vi "Align with Gear Peg.vi"(0 "Targets Message":T5={"type"="", "message"={"capturedAgoMs"=0, "targets"=[{"x"=0.0, "y"=0.0, "z"=0.0, "theta"=0.0}]}}, 1 "Swerve DevRef":T1[](array[typedef]), 2 "Wheel DevRef":T1[](array[typedef]), 3 "error in":errorcluster) -> (4 "Wheel Speed":dbl[](array[numeric]), 5 "Reverse?":bool[](array[boolean]), 6 "Swerve Speed":dbl[](array[numeric]), 7 "Setpoint":dbl[](array[numeric]), 8 "error out":errorcluster)   [LabVIEW 2016]
uses:
  Vision/Messages/Targets/Targets Message.ctl
  Vision/Messages/Targets/Targets Info.ctl
  <vilib>/Rock Robotics/WPI/MotorControl/WPI_MotorControlDeviceRef.ctl
  <vilib>/Rock Robotics/WPI/MotorControl/WPI_MotorControlType.ctl
  <vilib>/Rock Robotics/SystemInterfaces/DIO/FPGA_DIOPWMChannel.ctl
  <vilib>/Rock Robotics/WPI/PWM/WPI_PWMDeadband.ctl
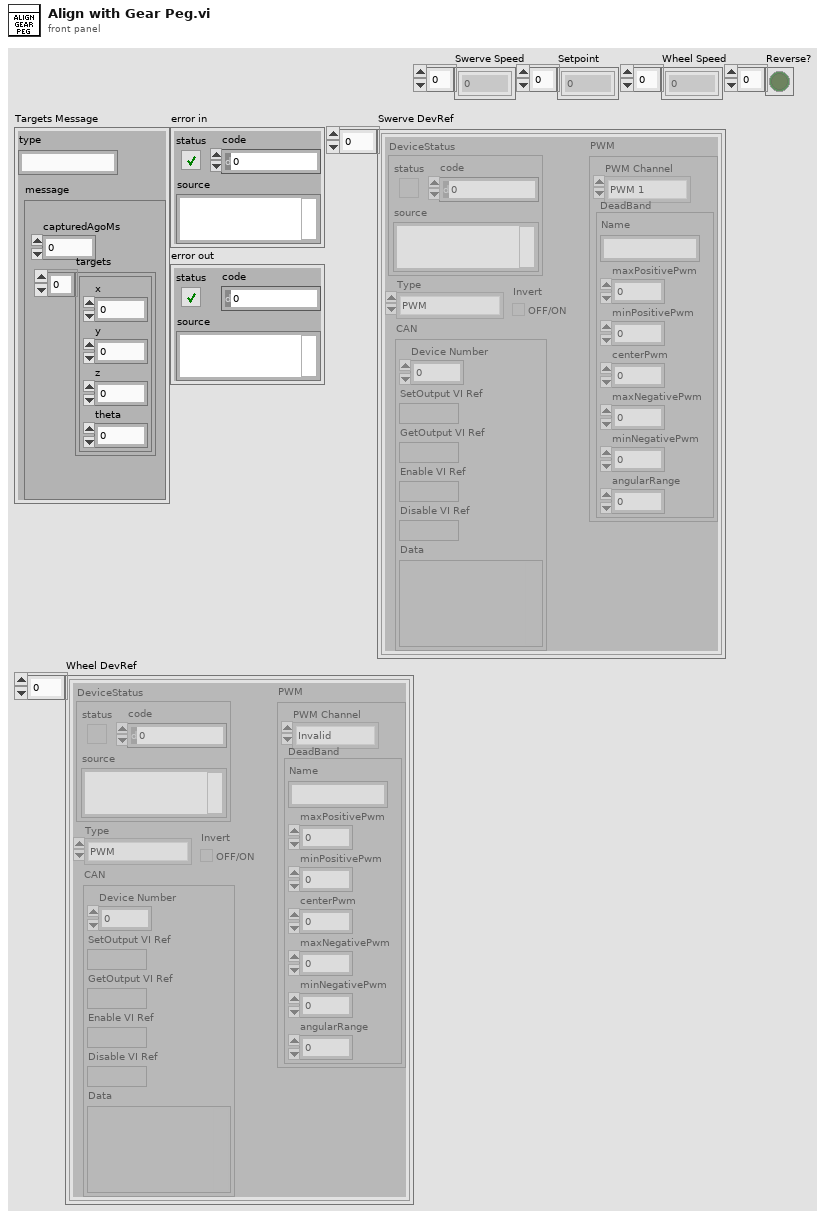
[diagram p1: front panel]
types:
  T1 = typedef "WPI_MotorControlDeviceRef.ctl" = cluster{"DeviceStatus":errorcluster, "Type":T2, "PWM":cluster{"PWM Channel":T3, "DeadBand":T4}, "CAN":cluster{"Device Number":u8, "SetOutput VI Ref":variant, "GetOutput VI Ref":variant, "Enable VI Ref":variant, "Disable VI Ref":variant, "Data":variant}, "Invert":bool}
  T2 = typedef "WPI_MotorControlType.ctl" = enum16{"PWM", "CAN"}
  T3 = typedef "FPGA_DIOPWMChannel.ctl" = enum8{"PWM 0", "PWM 1", "PWM 2", "PWM 3", "PWM 4", "PWM 5", "PWM 6", "PWM 7", "PWM 8", "PWM 9", "PWM MXP 0", "PWM MXP 1", "PWM MXP 2", "PWM MXP 3", "PWM MXP 4", "PWM MXP 5", "PWM MXP 6", "PWM MXP 7", "PWM MXP 8", "PWM MXP 9", "Invalid"}
  T4 = typedef "WPI_PWMDeadband.ctl" = cluster{"Name":string, "maxPositivePwm":i32, "minPositivePwm":i32, "centerPwm":i32, "maxNegativePwm":i32, "minNegativePwm":i32, "angularRange":u16}
  T5 = typedef "Targets Message.ctl" = cluster{"type":string, "message":cluster{"capturedAgoMs":i32, "targets":T6[]}}
  T6 = typedef "Targets Info.ctl" = cluster{"x":dbl, "y":dbl, "z":dbl, "theta":dbl}
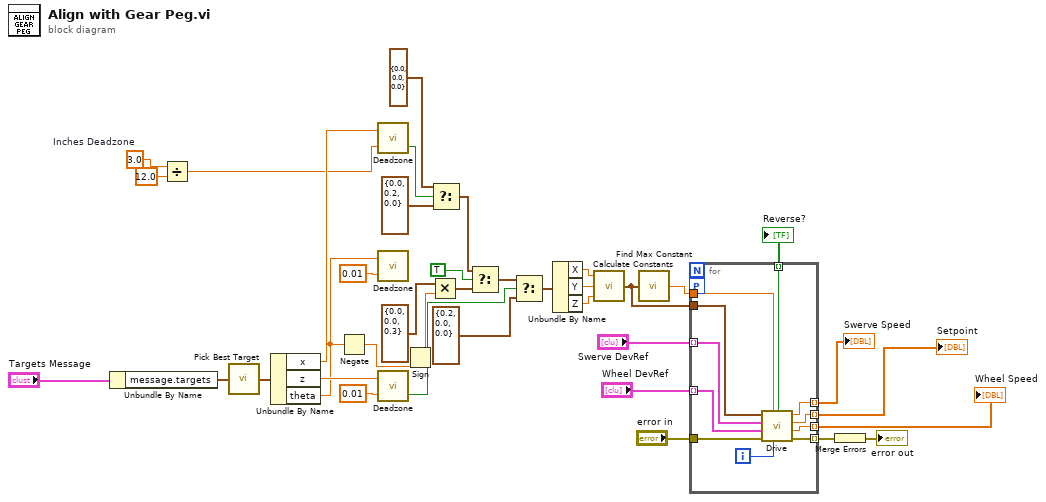
[diagram p0: block diagram]
diagram:
  w5 = 3.0  # Inches Deadzone
  n1 = Unbundle By Name("Targets Message") -> ("message.targets"=w37:T6[])
  n2 = Divide(x=w5, y=12.0) -> (x/y=w3:dbl)
  n3 = call "Pick Best Target.vi"("Target Infos"=w37) -> ("Best Target Info"=w36:T6)
  n4 = Unbundle By Name(w36) -> ("x"=w17:dbl, "z"=w23:dbl, "theta"=w20:dbl)
  n5 = Negate(x=w20) -> (-x=w21:dbl)
  n6 = call "Deadzone.vi"("Deadzone"=w3, "Value"=w17) -> ("In Deadzone?"=w32:bool)  [unwired: 1 out]
  n7 = call "Deadzone.vi"("Deadzone"=0.01, "Value"=w20) -> ()  [unwired: 2 out]
  n8 = call "Deadzone.vi"("Deadzone"=0.01, "Value"=w23) -> ("In Deadzone?"=w26:bool)  [unwired: 1 out]
  n9 = Sign(1:w21) -> (0:w1:dbl)
  n10 = Multiply(x=cluster{"X":dbl, "Y":dbl, "Z":dbl} {"X"=0.0, "Y"=0.0, "Z"=0.3}, y=w1) -> (x*y=w18:cluster{"X":dbl, "Y":dbl, "Z":dbl})
  n11 = Select(t=cluster{"X":dbl, "Y":dbl, "Z":dbl} {"X"=0.0, "Y"=0.0, "Z"=0.0}, s=w32, f=cluster{"X":dbl, "Y":dbl, "Z":dbl} {"X"=0.0, "Y"=0.2, "Z"=0.0}) -> (s? t:f=w25:cluster{"X":dbl, "Y":dbl, "Z":dbl})
  n12 = Select(t=w25, s=TRUE, f=w18) -> (s? t:f=w27:cluster{"X":dbl, "Y":dbl, "Z":dbl})
  n13 = Select(t=w27, s=w26, f=cluster{"X":dbl, "Y":dbl, "Z":dbl} {"X"=0.2, "Y"=0.0, "Z"=0.0}) -> (s? t:f=w31:cluster{"X":dbl, "Y":dbl, "Z":dbl})
  n14 = Unbundle By Name(w31) -> ("X"=w30:dbl, "Y"=w29:dbl, "Z"=w28:dbl)
  n15 = call "Calculate Constants.vi"("Z"=w28, "Y"=w29, "X"=w30) -> ("constants cluster"=w15:cluster{"a":dbl, "b":dbl, "c":dbl, "d":dbl})
  n16 = call "Find Max Constant.vi"("constants"=w15) -> ("Max or 1"=w14:dbl)
  n17 = for {
    tunnel: "Swerve DevRef" -> [w49] mode=indexing
    tunnel: w15 -> [w48]
    tunnel: w14 -> [w47]
    tunnel: "error in" -> [w45]
    tunnel: [w44] -> w12 mode=indexing
    tunnel: [w43] -> w9 mode=indexing
    tunnel: [w42] -> w8 mode=indexing
    tunnel: [w41] -> w7 mode=indexing
    tunnel: "Wheel DevRef" -> [w40] mode=indexing
    tunnel: [w39] -> w6 mode=indexing
    workers-P: _ -> [_]
    i -> [w46]
    n18 = call "Drive.vi"("Index"=w46, "Max Speed or 1"=w47, "error in"=w45, "Wheel DevRef"=w40, "Swerve DevRef"=w49, "constants"=w48) -> ("error out"=w44:errorcluster, "Wheel Speed"=w41:dbl, "Setpoint"=w42:dbl, "Swerve Speed"=w43:dbl, "Reverse?"=w39:bool)  [unwired: 1 in]
  }
  "Swerve Speed" <- w9
  "Setpoint" <- w8
  "Wheel Speed" <- w7
  "Reverse?" <- w6
  n19 = Merge Errors(w12) -> (→"error out":errorcluster)
